vi "tutte_le_guerre.vi"() -> ()   [LabVIEW 2013]
panel:
  in  "carri difesa":i32=5
  in  "carri attacco":i32=20
  out "Waveform Graph":i32[](graph)
  out "vittorie Jakuzia":i32
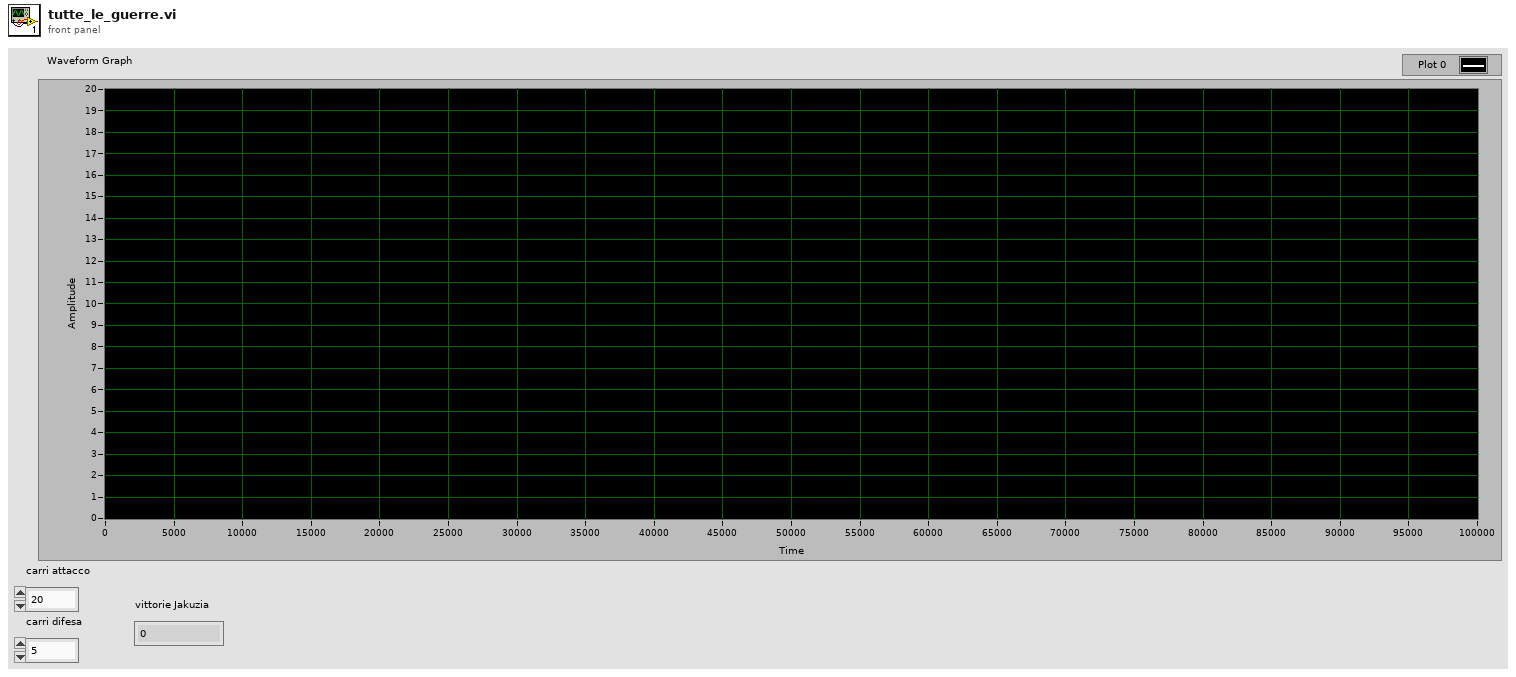
[diagram p1: front panel]
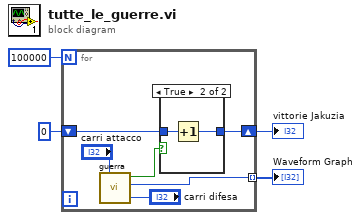
[diagram p0: block diagram]
diagram:
  n1 = for {
    N: 100000 -> [_]
    shift-right: [w9] -> w2
    shift-left: 0 -> [w10]
    tunnel: [w6] -> w1 mode=indexing
    n2 = call "guerra.vi"("carri difesa"="carri difesa", "carri attacco"="carri attacco") -> ("carri attacco\nrimanenti"=w6:i32, "attacco perde"=w5:bool)  [unwired: 7 in, 1 out]
    n3 = case shown="True" w5 {
      tunnel: w10 -> [w11 w13]
      tunnel: [w11 w12] -> w9
      frame False {
      }
      frame True {
        n4 = Increment(x=w13) -> (x+1=w12:i32)
      }
    }
  }
  "vittorie Jakuzia" <- w2
  "Waveform Graph" <- w1
